vi "State_Machine.vi"(8 "error in (no error)":errorcluster caption="entrée d'erreur (pas d'erreur)", 11 "Generate_SN en entrée":refnum<class "Generate_ID_Product_Nodon.lvclass">) -> (0 "error out":errorcluster caption="sortie d'erreur", 2 "Json_String":string, 3 "Generate_SN en sortie":refnum<class "Generate_ID_Product_Nodon.lvclass">)   [LabVIEW 2020, in "Library Test.lvlib" / "Generate_ID_Product_Nodon.lvclass"]
uses:
  Generate_ID_Product_Nodon.lvclass
  C:/Users/ngarcin/OneDrive - Altyor/Standard TB/Suite TB45/Class/Test/Test (Default)/Test (Default).lvclass
  Commun VI/TypeDef/Variable Printable.ctl
  JSON API/JSON Value/Set from JSON string.vi
  JSON API/JSON Value/JSON Value.lvclass
  JSON API/Variant JSON/Variant JSON.lvlib
  JSON API/Get Polymorphic/JSON GetSet.lvlib
  Commun VI/Library Commun.lvlib
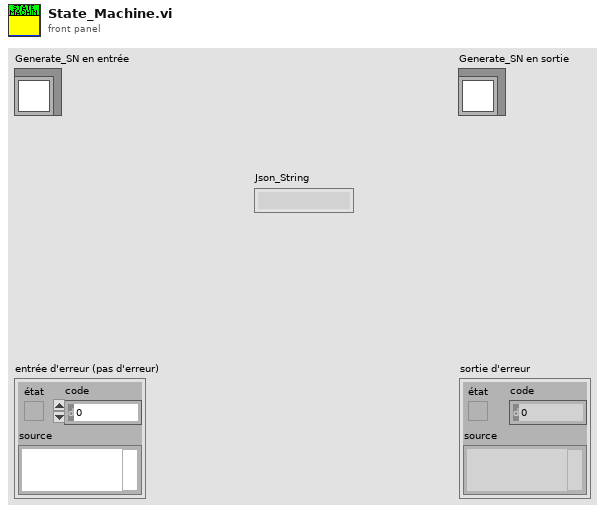
[diagram p1: front panel]
types:
  T1 = typedef "Variable Printable.ctl" = string
  T2 = enum16{"Get Variable", "Get All Variables", "Set Variable", "Delete Variable", "Delete All Variable"}
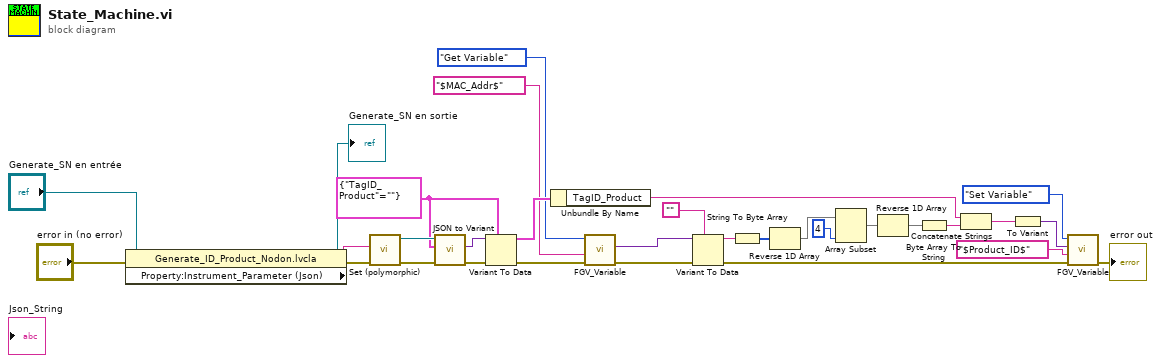
[diagram p0: block diagram]
diagram:
  w19 = cluster{"TagID_Product":string} {"TagID_Product"=""}
  n1 = property class="Generate_ID_Product_Nodon.lvcla"(reference="Generate_SN en entrée", error in="error in (no error)") -> (reference out=→"Generate_SN en sortie":refnum<class "Generate_ID_Product_Nodon.lvclass">, error out=w24:errorcluster, "Property:Instrument_Parameter (Json)"=w18:string)
  n2 = call-poly "Set (polymorphic).vi"("error in (no error)"=w24, "JSON stream"=w18) -> ("error out"=w26:errorcluster, "JSON Value out"=w28:refnum<class "JSON Value.lvclass">)  [unwired: 7 in, 1 out]
  n3 = call "JSON to Variant.vi"("error in (no error)"=w26, "Variant (Data Type)"=w19, "JSON Value"=w28) -> ("error out"=w27:errorcluster, "Variant out"=w25:variant)  [unwired: 7 in]
  n4 = Variant To Data(error in=w27, type=w19, Variant=w25) -> (data=w23:cluster{"TagID_Product":string}, error out=w16:errorcluster)
  n5 = Unbundle By Name(w23) -> ("TagID_Product"=w2:string)
  n6 = call "FGV_Variable.vi"("error in (no error)"=w16, "Variable"=T1 "$MAC_Addr$", "Function"=T2."Get Variable") -> ("error out"=w15:errorcluster, "Data Out"=w11:variant)  [unwired: 6 in, 1 out]
  n7 = Variant To Data(error in=w15, type="", Variant=w11) -> (data=w9:string, error out=w12:errorcluster)
  n8 = String To Byte Array(string=w9) -> (unsigned byte array=w8:u8[])
  n9 = Reverse 1D Array(array=w8) -> (reversed array=w7:u8[])
  n10 = Array Subset(array=w7, length=4 ("longueur")) -> (w5:u8[])  [unwired: 1 in]
  n11 = Reverse 1D Array(array=w5) -> (reversed array=w4:u8[])
  n12 = Byte Array To String(unsigned byte array=w4) -> (string=w3:string)
  n13 = Concatenate Strings(w2, w3) -> (w1:string)
  n14 = To Variant(anything=w1) -> (Variant=w20:variant)
  n15 = call "FGV_Variable.vi"("error in (no error)"=w12, "Variable"=T1 "$Product_ID$", "Data In"=w20, "Function"=T2."Set Variable") -> ("error out"=→"error out":errorcluster)  [unwired: 5 in, 2 out]
